vi "SubVI_Logfile.vi"(7 "Title":string, 8 "error in":errorcluster caption="err in", 11 "desc":string) -> (0 "error out":errorcluster caption="err out")   [LabVIEW 2016]
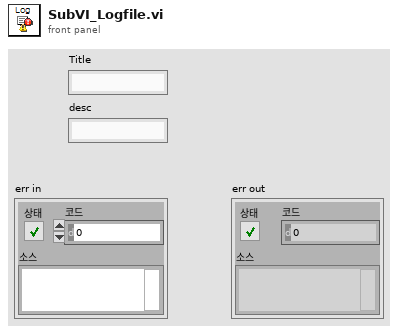
[diagram p1: front panel]
types:
  T1 = enum16{"open", "replace", "create", "open or create", "replace or create", "replace or create with confirmation"}
  T2 = cluster{"Test Information":cluster{"date":string, "custom":string, "oper":string, "package":string, "pkg side":string, "solder":string, "brd side":string, "paste":string, "reflow":string}, "Sensor Set":cluster{"Accelerometer":cluster{"Sensitivity(mV/g)":dbl}, "Strain Guage":cluster{"Ch.":dbl[], "Gage factor":dbl[], "Resistance":dbl[], "Poisson ratio":dbl[]}}, "Resistor Set":cluster{"Criterion Level":dbl, "Res. Set":cluster{"Res. Ch":dbl, "Res. Active":bool, "Res Initial":dbl}[]}, "Test Stop Condition":cluster{"Test cycle":u16, "Fail number in a cycle":u16, "Fail factor":cluster{"Duration":u16, "Fail No.":u16}}, "Acceleration Condition ":cluster{"Shock duration pecent [%]":u16, "Filter cutoff freq":u32}, "Save":cluster{"Save Path":path, "File Name":string}}
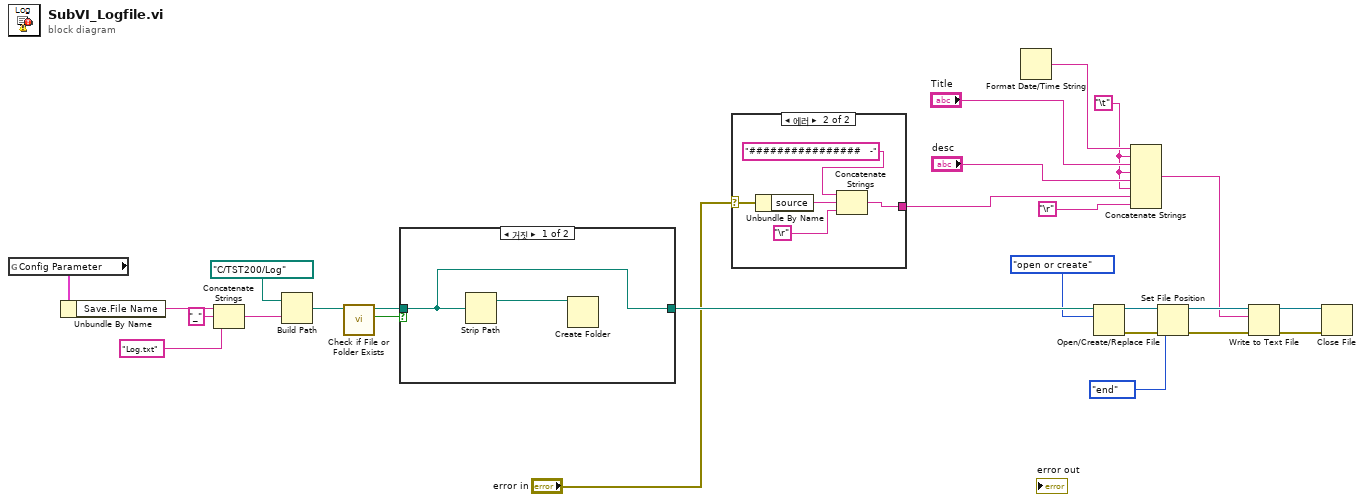
[diagram p0: block diagram]
diagram:
  w1 = "\t"
  n1 = global read "글로벌_Config Parameter.vi" "Config Parameter"() -> (w22:T2)
  n2 = Unbundle By Name(w22) -> ("Save.File Name"=w26:string)
  n3 = Concatenate Strings(w26, "_" ("문자열"), "Log.txt" ("문자열")) -> (w25:string)
  n4 = Build Path(base path=path "C:/TST200/Log" ("XML File Path"), name or relative path=w25) -> (appended path=w20:path)
  n5 = call <vilib>:"Check if File or Folder Exists.vi"("path"=w20) -> ("file or folder exists?"=w19:bool, "dup path"=w8:path)  [unwired: 8 in, 1 out]
  n6 = case shown="거짓" w19 {
    tunnel: w8 -> [w27 w29]
    tunnel: [w27 w29] -> w7
    frame False {
      n7 = Strip Path(path=w27) -> (stripped path=w28:path)  [unwired: 1 out]
      n8 = Create Folder(path (use dialog)=w28) -> ()  [unwired: 2 in, 3 out]
    }
    frame True {
    }
  }
  n9 = case shown="에러" "error in" {
    selector: "error in" -> [_ w34]
    tunnel: [_ w31] -> w4
    frame No Error {
    }
    frame Error {
      n10 = Unbundle By Name(w34) -> ("source"=w33:string)
      n11 = Concatenate Strings("################   -" ("문자열"), w33, "\r") -> (w31:string)
    }
  }
  n12 = Format Date/Time String() -> (date/time string=w11:string)  [unwired: 3 in]
  n13 = Open/Create/Replace File(file path (use dialog)=w7, operation (0:open)=T1."open or create" ("동작(0:open)")) -> (refnum out=w14:refnum<file>, error out=w17:errorcluster)  [unwired: 4 in, 1 out]
  n14 = Concatenate Strings(w11, w1, "Title", w1, "desc", w1, w4, "\r") -> (w3:string)
  n15 = Set File Position(refnum=w14, from (0:start)=enum16{"start", "end", "current"}."end" ("시작(0:시작)"), error in=w17) -> (refnum out=w15:refnum<file>, error out=w16:errorcluster)  [unwired: 1 in]
  n16 = Write to Text File(file (use dialog)=w15, text=w3, error in=w16) -> (refnum out=w12:refnum<file>, error out=w13:errorcluster)  [unwired: 1 in, 1 out]
  n17 = Close File(refnum=w12, error in=w13) -> ()  [unwired: 2 out]
